vi "SaveAs Document.vi"(8 "error in (no error)":errorcluster, 10 "Document Path":path, 11 "Document in":refnum<class "npoiDocument.lvclass">) -> (0 "error out":errorcluster, 3 "Document out":refnum<class "npoiDocument.lvclass">)   [LabVIEW 2017, in "NPOI_Document.lvlib" / "npoiDocument.lvclass"]
doc: "Saves the <b>Document</b> to the given <b>Document Path</b>.\n\nNotes:\n - If <b>Document Path</b> is empty (default) or is <Not A Path> or is a directory, the VI displays a dialog box from which the user can select a file. Error 43 occurs if you cancel the dialog box. \n - If the <b>Document Path</b> already contains a docuement with the same name then that file is overwritten without warning."
uses:
  npoiDocument.lvclass
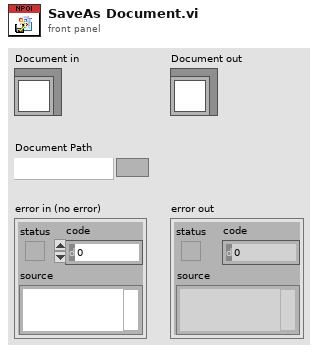
[diagram p1: front panel]
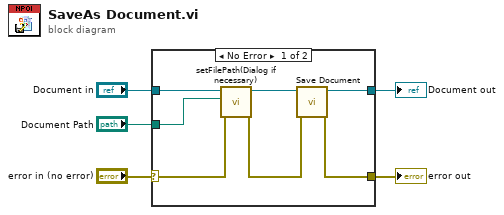
[diagram p0: block diagram]
diagram:
  n1 = case shown="No Error" "error in (no error)" {
    selector: "error in (no error)" -> [w10 w14]
    tunnel: [w7 w14] -> w4
    tunnel: [w6 w13] -> w2
    tunnel: "Document in" -> [w12 w13]
    tunnel: "Document Path" -> [w11 _]
    frame No Error {
      n2 = call "setFilePath(Dialog if necessary).vi"("error in (no error)"=w10, "File Path"=w11, "npoiDocument in"=w12) -> ("error out"=w8:errorcluster, "npoiDocument out"=w9:refnum<class "npoiDocument.lvclass">)  [unwired: 7 in]
      n3 = call "Save Document.vi"("error in (no error)"=w8, "Document in"=w9) -> ("error out"=w7:errorcluster, "Document out"=w6:refnum<class "npoiDocument.lvclass">)  [unwired: 8 in]
    }
    frame Error {
    }
  }
  "error out" <- w4
  "Document out" <- w2
